vi "MessageReceiver.vi"(0 "STOMP In":refnum<class "STOMP.lvclass">, 5 "error in (no error)":errorcluster) -> (19 "error out":errorcluster)   [LabVIEW 2017, in "LabVIEW STOMP.lvlib" / "STOMP.lvclass"]
uses:
  STOMP.lvclass
  STOMP.lvclass/STOMP.ctl
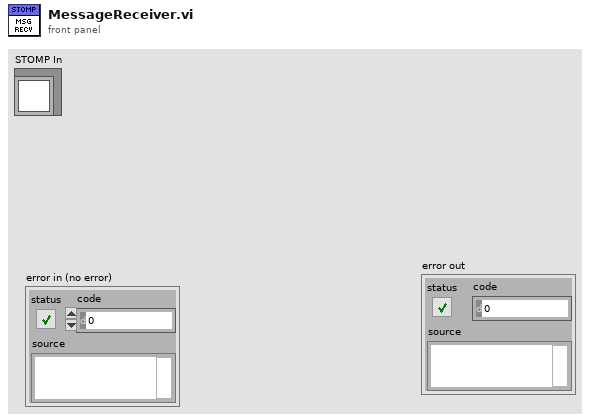
[diagram p1: front panel]
types:
  T1 = enum16{"Standard", "Buffered", "CRLF", "Immediate"}
  T2 = typedef "LabVIEW STOMP.lvlib/STOMP.lvclass/Type_ServerFrame.ctl" = cluster{"Type":T3, "Headers":cluster{"Header":string, "Value":string}[], "Body":string}
  T3 = typedef "LabVIEW STOMP.lvlib/STOMP.lvclass/Type_ServerFrameType.ctl" = enum16{"Undefined", "MESSAGE", "CONNECTED", "RECEIPT", "ERROR"}
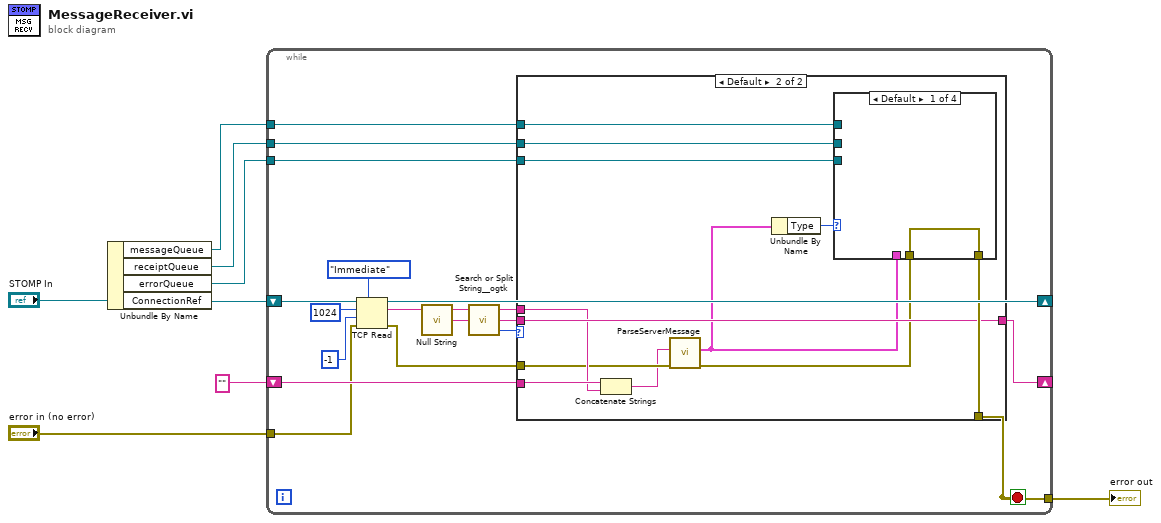
[diagram p0: block diagram]
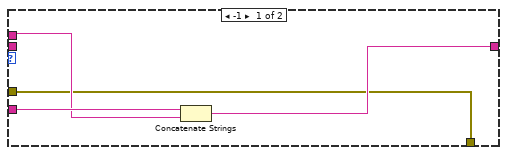
[diagram p2: hidden frame]
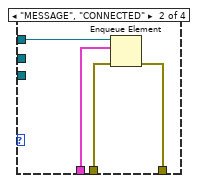
[diagram p3: hidden frame]
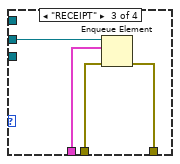
[diagram p4: hidden frame]
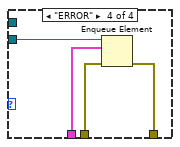
[diagram p5: hidden frame]
diagram:
  n1 = Unbundle By Name("STOMP In") -> ("messageQueue"=w3:refnum<queue>, "receiptQueue"=w2:refnum<queue>, "errorQueue"=w1:refnum<queue>, "ConnectionRef"=w6:refnum<k5>)
  n2 = while {
    shift-right: [w23] -> _
    shift-left: w6 -> [w24]
    shift-right: [w11] -> _
    shift-left: "" -> [w21]
    tunnel: w3 -> [w20]
    tunnel: "error in (no error)" -> [w18]
    tunnel: [w17] -> w4
    tunnel: w2 -> [w10]
    tunnel: w1 -> [w9]
    stop <- w17 stop-if-true
    n3 = TCP Read(connection ID=w24, bytes to read=1024, error in (no error)=w18, 7:T1."Immediate" ("mode (standard)"), 9:-1 ("timeout ms (25000)")) -> (connection ID out=w23:refnum<k5>, data out=w22:string, error out=w19:errorcluster)
    n4 = call "Null String.vi"() -> ("NULL"=w15:string)  [unwired: 19 in]
    n5 = call <userlib>:"Search or Split String__ogtk.vi"("search string/char (-)"=w15, "string"=w22) -> ("offset after match"=w13:i32, "substring after match"=w12:string, "substring before match"=w14:string)  [unwired: 1 in]
    n6 = case shown="Default" w13 {
      tunnel: w21 -> [w30 w42]
      tunnel: w20 -> [_ w41]
      tunnel: w19 -> [w27 w37]
      tunnel: [w27 w40] -> w17
      tunnel: w14 -> [w29 w38]
      tunnel: w12 -> [_ w39]
      tunnel: [w28 w39] -> w11
      tunnel: w10 -> [_ w33]
      tunnel: w9 -> [_ w32]
      frame -1 {
        n7 = Concatenate Strings(w30, w29) -> (w28:string)
      }
      frame Default {
        n8 = Concatenate Strings(w42, w38) -> (w36:string)
        n9 = call "ParseServerMessage.vi"("error in (no error)"=w37, "msg"=w36) -> ("error out"=w35:errorcluster, "ServerFrame"=w31:T2)  [unwired: 8 in]
        n10 = Unbundle By Name(w31) -> ("Type"=w34:T3)
        n11 = case shown="Default" w34 {
          tunnel: w41 -> [_ w47 _ _]
          tunnel: [w43 w46 w51 w55] -> w40
          tunnel: w35 -> [w43 w45 w50 w54]
          tunnel: w33 -> [_ _ w49 _]
          tunnel: w32 -> [_ _ _ w53]
          tunnel: w31 -> [_ w44 w48 w52]
          frame Default {
          }
          frame "MESSAGE", "CONNECTED" {
            n12 = Enqueue Element(queue=w47, element=w44, error in (no error)=w45) -> (error out=w46:errorcluster)  [unwired: 1 in, 2 out]
          }
          frame "RECEIPT" {
            n13 = Enqueue Element(queue=w49, element=w48, error in (no error)=w50) -> (error out=w51:errorcluster)  [unwired: 1 in, 2 out]
          }
          frame "ERROR" {
            n14 = Enqueue Element(queue=w53, element=w52, error in (no error)=w54) -> (error out=w55:errorcluster)  [unwired: 1 in, 2 out]
          }
        }
      }
    }
  }
  "error out" <- w4
